vi "CPP_ExponentialDecayFitDevelopment.vi"(4 "MedianFilter(points)":i32=3, 5 "SamplingRate":dbl, 6 "DecayData":dbl[](array[numeric]), 7 "FID ID":string) -> (0 "PlugInValues":string[](array[string]), 1 "smoothedCluster":T2, 2 "GraphClusterArray":T1(array[cluster]), 3 "PlugInTitles":string[](array[string]))   [LabVIEW 2012]
uses:
  <vilib>/addons/Time Series Analysis/Series Preprocess.llb/TSA Moving Average (Array).vi
  <vilib>/Analysis/baseanly.llb/Mean (DBL).vi
  <vilib>/Analysis/NI_AALPro.lvlib
  <vilib>/Analysis/NI_AALBase.lvlib
  <vilib>/addons/_Advanced Signal Processing/NI_AdvSigProcTSA.lvlib
panel:
  in  "End":dbl[](array[numeric])=[5.0, 15.0, 35.0]
  in  "Start":dbl[](array[numeric])=[3.0, 5.0, 15.0]
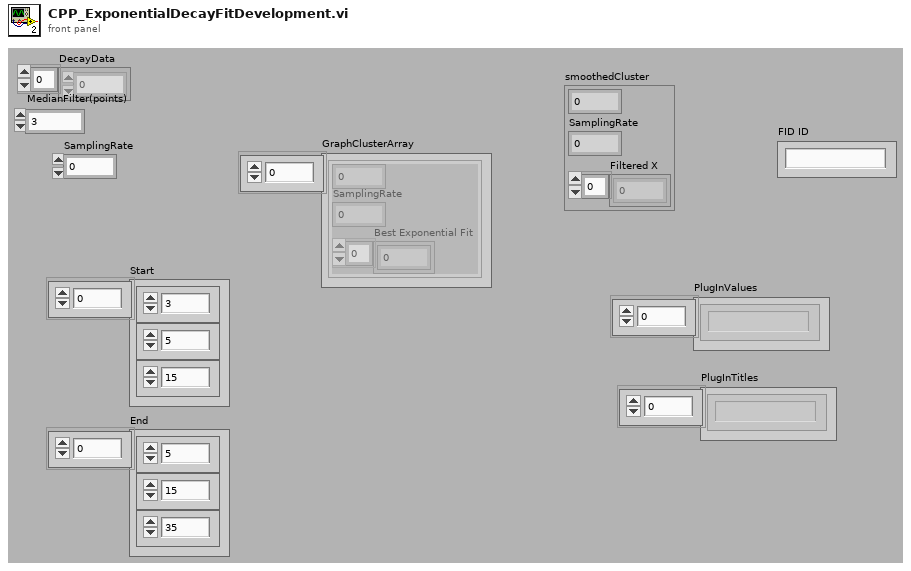
[diagram p1: front panel]
types:
  T1 = cluster{dbl, "SamplingRate":dbl, "Best Exponential Fit":dbl[]}[]
  T2 = cluster{"x*y":dbl, "SamplingRate":dbl, "Filtered X":dbl[]}
  T3 = cluster{dbl, "SamplingRate":dbl, "Best Exponential Fit":dbl[]}
  T4 = cluster{"x*y":dbl, "SamplingRate":dbl, "Xt out":dbl[]}
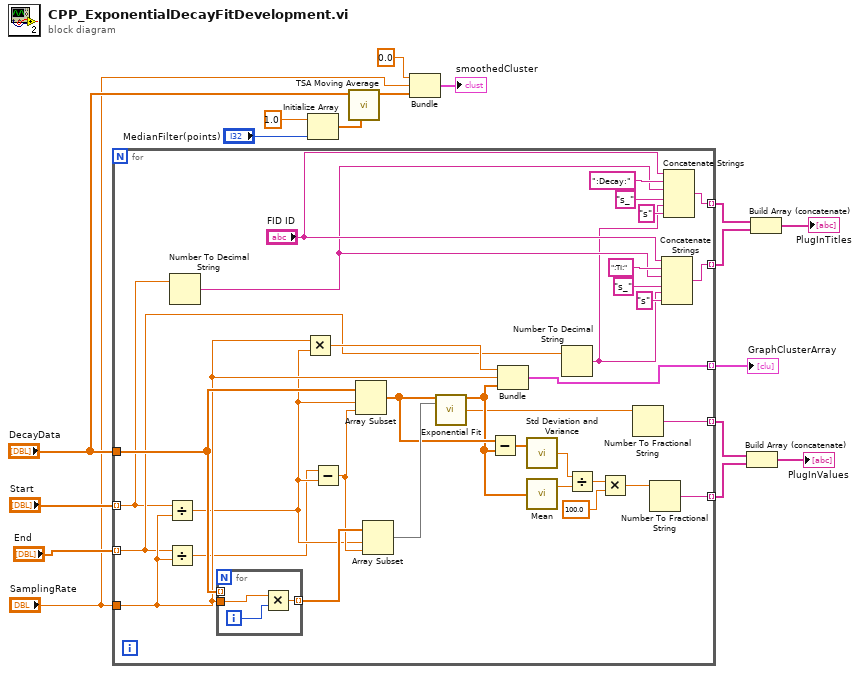
[diagram p0: block diagram]
diagram:
  n1 = for {
    tunnel: [w46] -> w7 mode=indexing
    tunnel: "DecayData" -> [w38]
    tunnel: "Start" -> [w18] mode=indexing
    tunnel: "SamplingRate" -> [w37]
    tunnel: "End" -> [w19] mode=indexing
    tunnel: [w20] -> w5 mode=indexing
    tunnel: [w21] -> w6 mode=indexing
    tunnel: [w24] -> w4 mode=indexing
    tunnel: [w22] -> w3 mode=indexing
    n2 = Divide(x=w18, y=w37) -> (x/y=w35:dbl)
    n3 = Divide(x=w19, y=w37) -> (x/y=w33:dbl)
    n4 = Number To Decimal String(number=w18) -> (decimal integer string=w27:string)  [unwired: 1 in]
    n5 = for {
      tunnel: w38 -> [_] mode=indexing
      tunnel: w37 -> [w52]
      tunnel: [w51] -> w50 mode=indexing
      i -> [w53]
      n6 = Multiply(x=w52, y=w53) -> (x*y=w51:dbl)
    }
    n7 = Multiply(x=w37, y=w35) -> (x*y=w47:dbl)
    n8 = Subtract(x=w33, y=w35) -> (x-y=w49:dbl)
    n9 = Array Subset(array=w38, index=w35, length=w49) -> (w45:dbl[])
    n10 = Array Subset(array=w50, index=w35, length=w49) -> (w48:dbl[])
    n11 = call <vilib>:"Exponential Fit.vi"("Y"=w45, "X"=w48) -> ("Best Exponential Fit"=w43:dbl[], "damping"=w25:dbl)  [unwired: 8 in, 4 out]
    n12 = Subtract(x=w45, y=w43) -> (x-y=w44:dbl[])
    n13 = Bundle(w47, "SamplingRate"=w37, "Best Exponential Fit"=w43) -> (w46:T3)  [unwired: 1 out]
    n14 = call <vilib>:"Std Deviation and Variance.vi"("X"=w44) -> ("standard deviation"=w42:dbl)  [unwired: 1 in, 2 out]
    n15 = call-poly <vilib>:"Mean.vi"("X"=w43) -> ("mean"=w41:dbl)  [unwired: 1 out]
    n16 = Number To Decimal String(number=w19) -> (decimal integer string=w26:string)  [unwired: 1 in]
    n17 = Divide(x=w42, y=w41) -> (x/y=w40:dbl)
    n18 = Multiply(x=w40, y=100.0) -> (x*y=w23:dbl)
    n19 = Number To Fractional String(number=w25) -> (F-format string=w24:string)  [unwired: 3 in]
    n20 = Number To Fractional String(number=w23) -> (F-format string=w22:string)  [unwired: 3 in]
    n21 = Concatenate Strings("FID ID", ":TI:" ("string"), w27, "s_" ("string"), w26, "s" ("string")) -> (w20:string)
    n22 = Concatenate Strings("FID ID", ":Decay:" ("string"), w27, "s_" ("string"), w26, "s" ("string")) -> (w21:string)
  }
  "GraphClusterArray" <- w7
  n23 = Initialize Array(1.0 ("element"), "MedianFilter(points)") -> (w14:dbl[])
  n24 = call-poly <vilib>:"TSA Moving Average.vi"("user defined weights"=w14, "Xt"="DecayData") -> ("Xt out"=w15:dbl[])  [unwired: 8 in, 1 out]
  n25 = Bundle("x*y"=0.0, "SamplingRate"="SamplingRate", "Xt out"=w15) -> (→"smoothedCluster":T4)  [unwired: 1 out]
  n26 = Build Array (concatenate)(w4, w3) -> (→"PlugInValues":string[])
  n27 = Build Array (concatenate)(w6, w5) -> (→"PlugInTitles":string[])
